vi "TxTestExample.vi"() -> ()   [LabVIEW 2014]
uses:
  PhyPort.ctl
  PhyType.ctl
  standard.ctl
  BW.ctl
  LegacyDataRate.ctl
  VISAOperation.ctl
panel:
  in  "AnalysisConfig":T6={"PortName"="WLAN_DUT0_ANT0", "PhyPort"=enum."Port5", "ExternalAtt"=0, "TriggerLevel"=-40, "NumberofChain"=1, "AcqLength"=0.0001, "MCSIndex"=7.0, "PhyType"=enum."VHT", "Standard"=enum."802.11 ac", "BW"=enum."80M", "TriggerSource"=enum."RIO0", "Freq"=5180000000.0, "LegacyDataRate"=enum."R1M"}
  out "Results":string[](array[string])=["1,-15.852258,-4.171936,-16.616194\n", "1,-32.7547,-33.0151,-32.7485\n", "-3.528785,-4.156985,0.733084,0.368447,1,0.021492,0.825732,-38.226673,0.000000\n", "1,7.960808,5299532163.742691,0.000000\n"]
  in  "VISA resource name":refnum<visa-resource-name>="TCPIP0::10.144.41.48::inst0::INSTR"
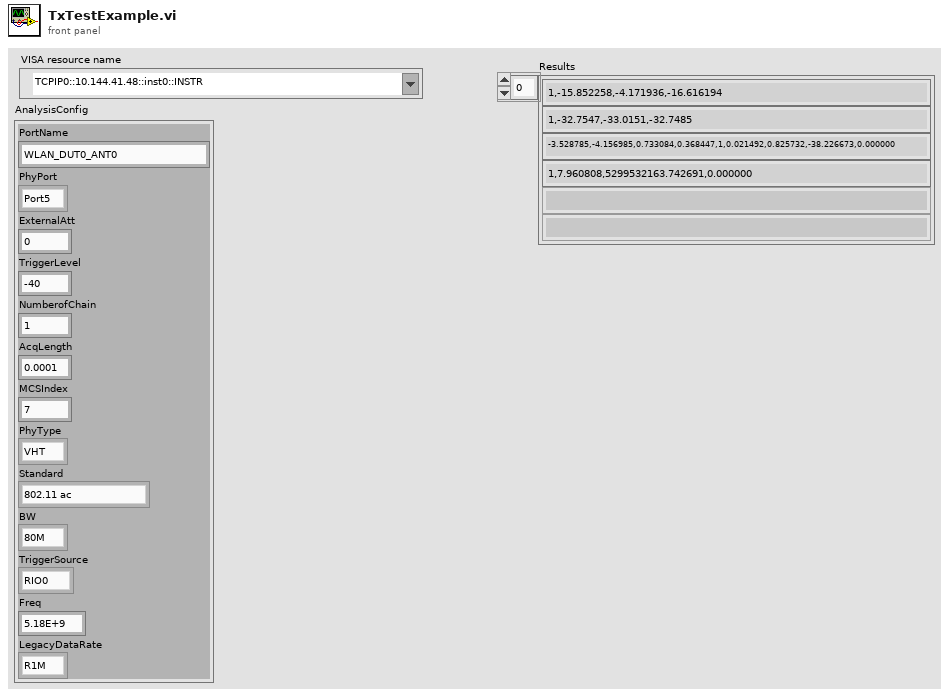
[diagram p1: front panel]
types:
  T1 = typedef "PhyPort.ctl" = enum16{"Port0", "Port1", "Port2", "Port3", "Port4", "Port5", "Port6", "Port7"}
  T2 = typedef "PhyType.ctl" = enum16{"DSSS", "OFDM", "HT", "VHT"}
  T3 = typedef "standard.ctl" = enum16{"802.11 a/g", "802.11 b/g", "802.11 g", "802.11 n", "802.11 ac"}
  T4 = typedef "BW.ctl" = enum16{"5M", "10M", "20M", "40M", "80M", "160M"}
  T5 = typedef "LegacyDataRate.ctl" = enum16{"R1M", "R2M", "R5M5", "R6M", "R9M", "R11M", "R12M", "R18M", "R24M", "R36M", "R48M", "R54M"}
  T6 = cluster{"PortName":string, "PhyPort":T1, "ExternalAtt":i32, "TriggerLevel":i32, "NumberofChain":i32, "AcqLength":dbl, "MCSIndex":dbl, "PhyType":T2, "Standard":T3, "BW":T4, "TriggerSource":enum16{"RIO0", "RIO1"}, "Freq":dbl, "LegacyDataRate":T5}
  T7 = typedef "VISAOperation.ctl" = enum16{"RunFile", "OpenDebugPanel", "ReadError", "ReadSTB", "Reset", "Clean", "CloseVISA", "RunCMD", "OpenVISA"}
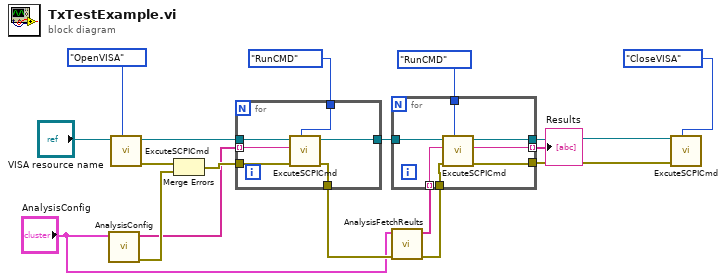
[diagram p0: block diagram]
diagram:
  n1 = call "AnalysisConfig.vi"("AnalysisConfig"="AnalysisConfig") -> ("error out"=w10:errorcluster, "AnalysisConfigCMD"=w2:string[])  [unwired: 9 in]
  n2 = call "ExcuteSCPICmd.vi"("VISAOperation"=VISAOperation."OpenVISA", "VISA resource name"="VISA resource name") -> ("error out"=w14:errorcluster, "reference out"=w13:refnum<visa-resource-name>)  [unwired: 6 in, 2 out]
  n3 = Merge Errors(w14, w10) -> (w9:errorcluster)
  n4 = for {
    tunnel: VISAOperation."RunCMD" ("VISAOperation") -> [w22]
    tunnel: w13 -> [w24]
    tunnel: [w23] -> w12
    tunnel: w2 -> [w21] mode=indexing
    tunnel: w9 -> [w20]
    tunnel: [w19] -> w8
    n5 = call "ExcuteSCPICmd.vi"("VISAOperation"=w22, "error in (no error)"=w20, "Run Command"=w21, "VISA resource name"=w24) -> ("error out"=w19:errorcluster, "reference out"=w23:refnum<visa-resource-name>)  [unwired: 4 in, 2 out]
  }
  n6 = call "AnalysisFetchReults.vi"("error in (no error)"=w8, "AnalysisConfig"="AnalysisConfig") -> ("error out"=w6:errorcluster, "FetchCMD"=w7:string[])  [unwired: 8 in]
  n7 = for {
    tunnel: VISAOperation."RunCMD" ("VISAOperation") -> [w31]
    tunnel: w12 -> [w30]
    tunnel: [w27] -> w5
    tunnel: w7 -> [w29] mode=indexing
    tunnel: w6 -> [w28]
    tunnel: [w26] -> w4
    tunnel: [w25] -> w3 mode=indexing
    n8 = call "ExcuteSCPICmd.vi"("VISAOperation"=w31, "error in (no error)"=w28, "Run Command"=w29, "VISA resource name"=w30) -> ("error out"=w26:errorcluster, "Results"=w25:string, "reference out"=w27:refnum<visa-resource-name>)  [unwired: 4 in, 1 out]
  }
  "Results" <- w3
  n9 = call "ExcuteSCPICmd.vi"("VISAOperation"=VISAOperation."CloseVISA", "error in (no error)"=w4, "VISA resource name"=w5) -> ()  [unwired: 5 in, 4 out]
